vi "CheckFaultConditions.vi"(0 "Array 2":cluster{"SensorCluster":T1}[](array[cluster]), 5 "DisableFaultCheck":bool, 7 "ControlState":T3(ring), 9 "?":T2) -> (4 "Array out":cluster{"SensorCluster":T1}[](array[cluster]), 6 "Fault?":bool)   [LabVIEW 2018]
uses:
  Type_Def/Master_DataControl.ctl
  Type_Def/TypeDef_cRIODatas.ctl
  Type_Def/Type_Def IMUDatas.ctl
  Type_Def/TypeDef_BMSDatas.ctl
  Type_Def/TypeDef_BMSStatuss.ctl
  Type_Def/TypeDef FixedMotorData.ctl
  Type_Def/Type_Def ClusterSensor.ctl
  Type_Def/Type_Def Actuator Controls.ctl
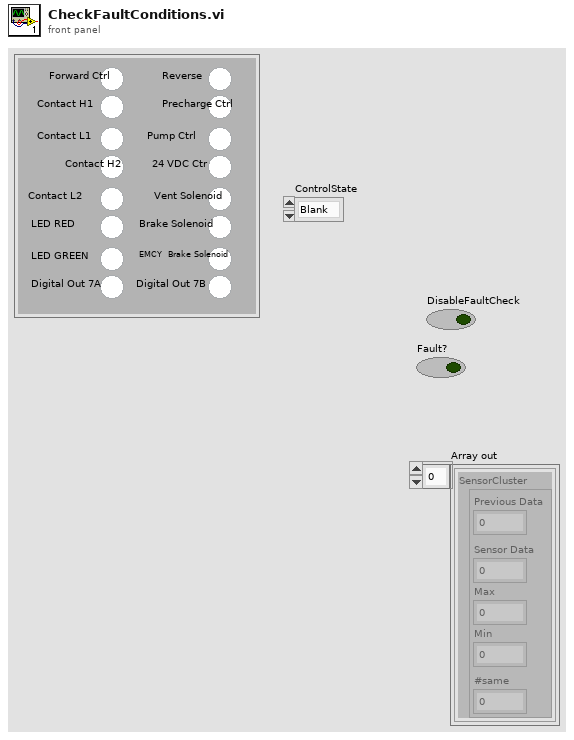
[diagram p1: front panel]
types:
  T1 = typedef "Type_Def ClusterSensor.ctl" = cluster{"Sensor Data":dbl, "Max":dbl, "Min":dbl, "Previous Data":dbl, "#same":dbl}
  T2 = typedef "Type_Def Actuator Controls.ctl" = cluster{"Reverse ":bool, "Precharge Ctrl":bool, "Pump Ctrl":bool, "24 VDC Ctr":bool, "Vent Solenoid":bool, "Brake Solenoid":bool, "EMCY  Brake Solenoid":bool, "Digital Out 7B ":bool, "Forward Ctrl":bool, "Contact H1":bool, "Contact L1":bool, "Contact H2":bool, "Contact L2 ":bool, "LED RED":bool, "LED GREEN":bool, " Digital Out 7A":bool}
  T3 = enum16{"Blank", "Systems Check", "Idle", "Ready", "Pushing", "CrawlingPrecharge", "Braking", "Fault", "Boot Up", "Unpowered", "Crawling", "Shutdown", "Service Push", "Service Wait", "Vent", "Precharge", "Cooldown"}
  T4 = typedef "Master_DataControl.ctl" = cluster{"cRIO Data":T5, "IMU Data":T6, "BMS Data":T7, "Motor Data":T9}
  T5 = typedef "TypeDef_cRIODatas.ctl" = cluster{"HallEffect Right (cm)":dbl, "HallEffect Left (cm)":dbl, "Optical Sensor 1 (V)":dbl, "Optical Sensor 2 (V)":dbl, "24V Voltage  (V)":dbl, "24V Current (A)":dbl, "Contactor H1 Continuity":dbl, "Contactor L1 Continuity ":dbl, "Contactor H2 Continuity":dbl, "Contactor L2 Continuity ":dbl, "Brake PT(psig)":dbl, "Pump PT (psig)":dbl, "24V Temp   (C)":dbl, "Tank PT(psig) ":dbl, "ABS Pressure 1 (psig)":dbl, "ABS Pressure 2 (psig) ":dbl, "Displacement (ft)":dbl, "Velocity (ft/s)":dbl, "Time (ms)":dbl}
  T6 = typedef "Type_Def IMUDatas.ctl" = cluster{"x acceleration (g)":dbl, "Pressure (psia)":dbl, "Temperature (F)":dbl}
  T7 = typedef "TypeDef_BMSDatas.ctl" = cluster{"Pack 1 Max Cell\n Voltage (V)":dbl, "Pack 1 Max Cell\n ID ":dbl, "Pack 1 Min Cell \nVoltage (V)":dbl, "Pack 1 Min Cell \nID ":dbl, "Pack 1 State of Charge  (%)":dbl, "Pack 1 Average Voltage1 (V)":dbl, "Pack 1Voltage Delta (V)":dbl, "Pack 1 Current (A)":dbl, "Pack 1 Voltage (V)":dbl, "Pack 1 Max Resistance (Ohm)":dbl, "Pack 1Min Resistance (Ohm)":dbl, "Pack 1Average Resistance (Ohm)":dbl, "Pack 1Delta Resistance (Ohm)":dbl, "Pack 1 Highest Temperature(F)":dbl, "BmsStatus":T8, "Pack 2 Max Cell\n Voltage (V) ":dbl, "Pack 2 Max Cell\n ID  ":dbl, "Pack 2 Min Cell \nVoltage (V) ":dbl, "Pack 2 Min Cell \nID  ":dbl, "Pack 2 Average Voltage1 (V)":dbl, "Pack 2 Voltage Delta (V) ":dbl, "Pack 2 Current (A)":dbl, "Pack 2 Voltage (V) ":dbl, "Pack 2 State of Charge  (%) ":dbl, "Pack 2 Max Resistance (Ohm) ":dbl, "Pack 2 Min Resistance (Ohm)":dbl, "Pack 2 Average Resistance (Ohm)":dbl, "Pack 2 Delta Resistance (Ohm) ":dbl, "Pack 2 Highest Temperature(F) ":dbl}
  T8 = typedef "TypeDef_BMSStatuss.ctl" = cluster{"isFault":bool, "isolationMonitoring":bool}
  T9 = typedef "TypeDef FixedMotorData.ctl" = cluster{" Velocity (RPM)":dbl, " MotorTemp(C)":dbl, " ControlTemp(C)":dbl, " DcLinkVolt(V)":dbl, " ErrorCode":dbl, "IsAlive":bool, "motorStatus":cluster{"isReady":bool, "isOn":bool, "isOperEn":bool, "isFault":bool, "isVoltEn":bool, "targetReached":bool, "isWarning":bool}, "motorControllerState":u16}
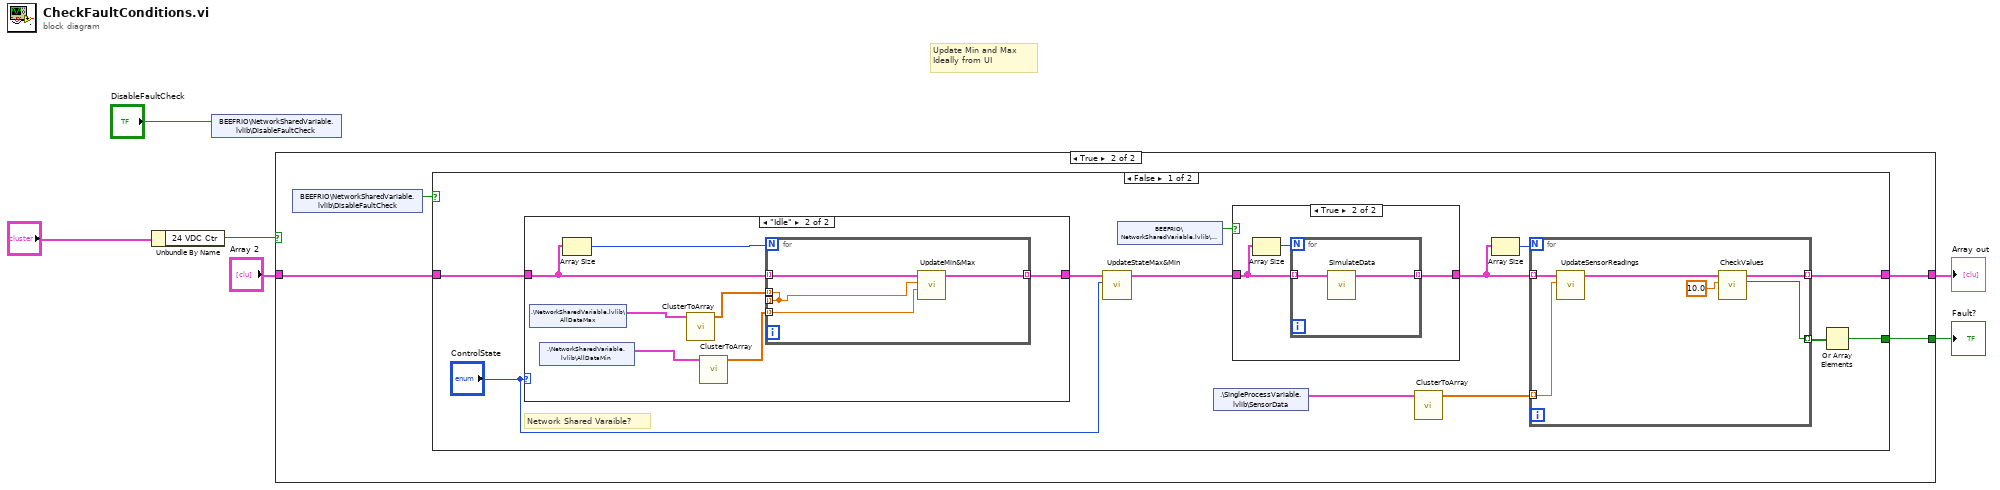
[diagram p0: block diagram]
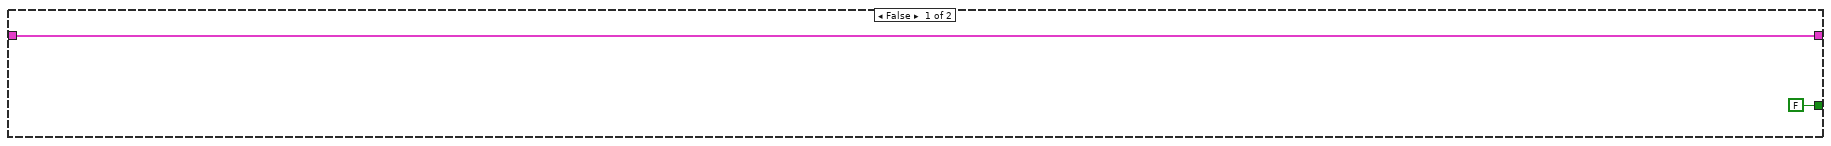
[diagram p2: hidden frame]
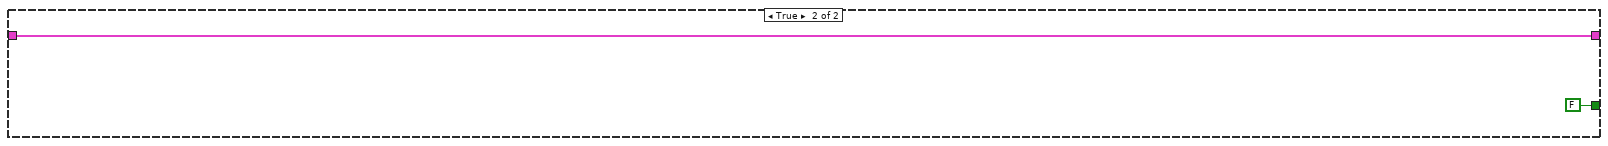
[diagram p5: hidden frame]
diagram:
  # "Update Min and Max \nIdeally from UI"
  n1 = Unbundle By Name("?") -> ("24 VDC Ctr"=w4:bool)
  n2 = shared-variable "BEEFRIO\\NetworkSharedVariable.lvlib\\DisableFaultCheck"("DisableFaultCheck") -> ()  [unwired: 1 in, 1 out]
  n3 = case shown="True" w4 {
    tunnel: [FALSE w10] -> w3
    tunnel: [w7 w11] -> w2
    tunnel: "Array 2" -> [w7 w9]
    frame False {
    }
    frame True {
      n4 = shared-variable "BEEFRIO\\NetworkSharedVariable.lvlib\\DisableFaultCheck"() -> (w12:bool)  [unwired: 1 in, 1 out]
      n5 = case shown="False" w12 {
        tunnel: w9 -> [w24 w50]
        tunnel: [w13 w50] -> w11
        tunnel: [w14 FALSE] -> w10
        frame False {
          # "Network Shared Varaible?"
          n6 = case shown="\"Idle\"" "ControlState" {
            tunnel: w24 -> [w37 w43]
            tunnel: [w37 w41] -> w18
            frame "Blank", Default {
            }
            frame "Idle" {
              n7 = shared-variable ".\\NetworkSharedVariable.lvlib\\AllDataMax"() -> (w39:T4)  [unwired: 1 in, 1 out]
              n8 = shared-variable ".\\NetworkSharedVariable.lvlib\\AllDataMin"() -> (w38:T4)  [unwired: 1 in, 1 out]
              n9 = Array Size(array=w43) -> (size(s)=w42:i32)
              n10 = call "ClusterToArray.vi"("SensorData"=w39) -> ("Array"=w40:dbl[])  [unwired: 9 in]
              n11 = call "ClusterToArray.vi"("SensorData"=w38) -> ("Array"=w44:dbl[])  [unwired: 9 in]
              n12 = for {
                N: w42 -> [_]
                tunnel: [w45] -> _ mode=indexing
                tunnel: w44 -> [w48] mode=indexing
                tunnel: [w46] -> w41 mode=indexing
                tunnel: w43 -> [w47] mode=indexing
                tunnel: w40 -> [w45] mode=indexing
                n13 = call "UpdateMin&Max.vi"("Numeric 24"=w48, "Numeric 25"=w45, "Cluster in"=w47) -> ("Cluster out"=w46:cluster{"SensorCluster":T1})  [unwired: 8 in]
              }
            }
          }
          n14 = call "UpdateStateMax&Min.vi"("ControlState"="ControlState", "Array in"=w18) -> ("Array out"=w21:cluster{"SensorCluster":T1}[])  [unwired: 9 in]
          n15 = shared-variable "BEEFRIO\\NetworkSharedVariable.lvlib\\SimulateData"() -> (w17:bool)  [unwired: 1 in, 1 out]
          n16 = shared-variable ".\\SingleProcessVariable.lvlib\\SensorData"() -> (w16:T4)  [unwired: 1 in, 1 out]
          n17 = case shown="True" w17 {
            tunnel: w21 -> [w25 w27]
            tunnel: [w25 w26] -> w22
            frame False {
            }
            frame True {
              n18 = Array Size(array=w27) -> (size(s)=w28:i32)
              n19 = for {
                N: w28 -> [_]
                tunnel: w27 -> [w30] mode=indexing
                tunnel: [w29] -> w26 mode=indexing
                n20 = call "SimulateData.vi"("Cluster in"=w30) -> ("Cluster out"=w29:cluster{"SensorCluster":T1})  [unwired: 10 in]
              }
            }
          }
          n21 = call "ClusterToArray.vi"("SensorData"=w16) -> ("Array"=w20:dbl[])  [unwired: 9 in]
          n22 = Array Size(array=w22) -> (size(s)=w19:i32)
          n23 = for {
            N: w19 -> [_]
            tunnel: [w35] -> w23 mode=indexing
            tunnel: [w34] -> w13 mode=indexing
            tunnel: w20 -> [w33] mode=indexing
            tunnel: w22 -> [w32] mode=indexing
            n24 = call "UpdateSensorReadings.vi"("Data in"=w33, "Cluster in"=w32) -> ("Cluster out"=w36:cluster{"SensorCluster":T1})  [unwired: 9 in]
            n25 = call "CheckValues.vi"("y"=10.0, "Cluster in"=w36) -> ("Boolean"=w35:bool, "Cluster out"=w34:cluster{"SensorCluster":T1})  [unwired: 8 in]
          }
          n26 = Or Array Elements(Boolean array=w23) -> (logical OR=w14:bool)
        }
        frame True {
        }
      }
    }
  }
  "Array out" <- w2
  "Fault?" <- w3
